vi "Get Data.vi"(8 "error in (no error)":errorcluster, 10 "Data Type":string, 11 "Communication in":refnum<class "Communication.lvclass">) -> (0 "error out":errorcluster, 3 "Communication out":refnum<class "Communication.lvclass">)   [LabVIEW 2021, in "Communication.lvclass"]
uses:
  Communication.lvclass
  Data/Data.lvclass
  Controls/User Event Operation.ctl
  Downloads/Sample PC Template/Sample PC Template/Typedefs/Data.ctl
  Downloads/Sample PC Template/Sample PC Template/Sample PC Template.lvlib
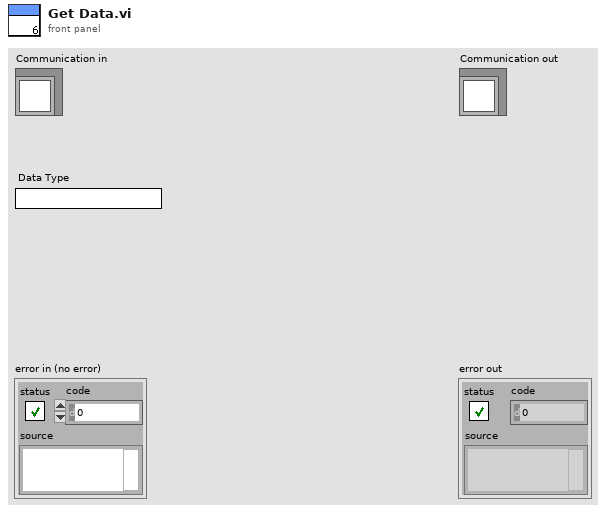
[diagram p1: front panel]
types:
  T1 = typedef "Sample PC Template.lvlib/Data.ctl" = cluster{"State":string, "Data":variant}
  T2 = typedef "User Event Operation.ctl" = enum16{"Obtain", "Generate", "Release"}
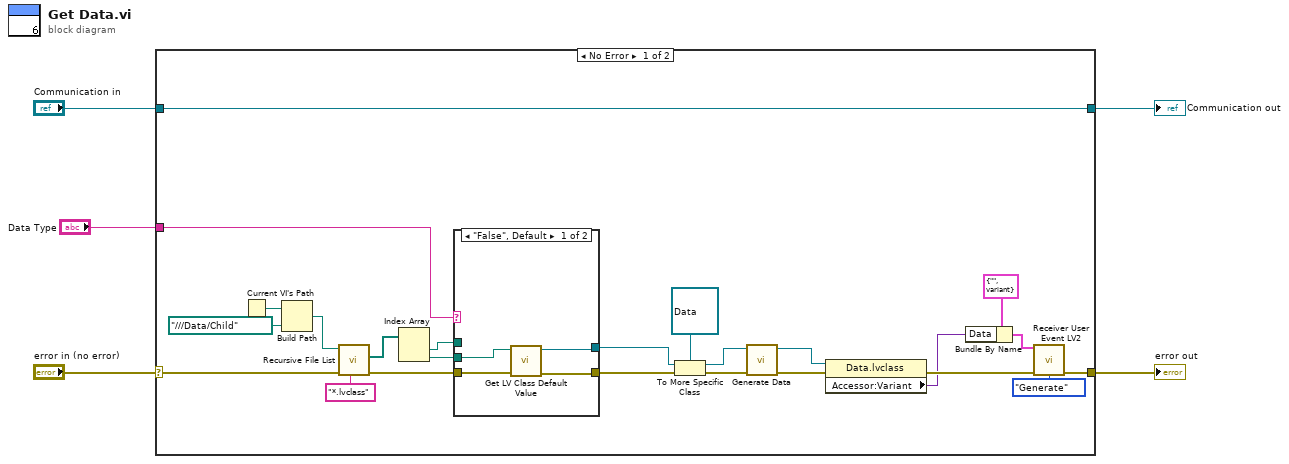
[diagram p0: block diagram]
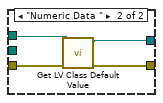
[diagram p2: hidden frame]
diagram:
  n1 = case shown="No Error" "error in (no error)" {
    selector: "error in (no error)" -> [w20 w39]
    tunnel: [w10 w39] -> w4
    tunnel: [w29 w38] -> w2
    tunnel: "Communication in" -> [w29 w38]
    tunnel: "Data Type" -> [w21 _]
    frame No Error {
      n2 = Current VI's Path() -> (path=w28:path)
      n3 = Build Path(base path=w28, name or relative path=path "../../../Data/Child") -> (appended path=w27:path)
      n4 = call <vilib>:"Recursive File List.vi"("pattern"="*.lvclass", "error in (no error)"=w20, "Folder Path"=w27) -> ("error out"=w25:errorcluster, "All Files in Dir"=w24:path[])  [unwired: 4 in, 3 out]
      n5 = Index Array(array=w24) -> (element #1=w23:path, element #2=w22:path)  [unwired: 2 in]
      n6 = case shown="\"False\", Default" w21 {
        tunnel: w25 -> [w33 w37]
        tunnel: [w30 w36] -> w18
        tunnel: w23 -> [_ w35]
        tunnel: [w31 w34] -> w16
        tunnel: w22 -> [w32 _]
        frame "False", Default {
          n7 = call <vilib>:"Get LV Class Default Value.vi"("error in (no error)"=w33, "class path"=w32) -> ("error out"=w30:errorcluster, "object"=w31:refnum<class>)  [unwired: 8 in]
        }
        frame "Numeric Data " {
          n8 = call <vilib>:"Get LV Class Default Value.vi"("error in (no error)"=w37, "class path"=w35) -> ("error out"=w36:errorcluster, "object"=w34:refnum<class>)  [unwired: 8 in]
        }
      }
      n9 = To More Specific Class(target class=refnum<class "Data.lvclass"> refnum ("Data.lvclass"), reference=w16, error in=w18) -> (specific class reference=w14:refnum<class "Data.lvclass">, error out=w15:errorcluster)
      n10 = call-dynamic "Generate Data.vi"("error in (no error)"=w15, "Data in"=w14) -> ("error out"=w13:errorcluster, "Data out"=w12:refnum<class "Data.lvclass">)  [unwired: 8 in]
      n11 = property class="Data.lvclass"(reference=w12, error in=w13) -> (error out=w11:errorcluster, "Accessor:Variant"=w7:variant)  [unwired: 1 out]
      n12 = Bundle By Name(cluster=T1 {"State"="", "Data"=variant} ("Data"), "Data"=w7) -> (w6:T1)
      n13 = call "Receiver User Event LV2.vi"("Data"=w6, "Error In"=w11, "Operation"=User_Event_Operation."Generate") -> ("Error Out"=w10:errorcluster)  [unwired: 11 in, 1 out]
    }
    frame Error {
    }
  }
  "error out" <- w4
  "Communication out" <- w2
